vi "2. QRcode.vi"() -> ()   [LabVIEW 2019]
uses:
  <vilib>/vision/Instrument.llb/QR Code Report.ctl
  <vilib>/vision/Instrument.llb/QR Code Model Type.ctl
  <vilib>/vision/Instrument.llb/QR Code Stream Mode Type.ctl
  <vilib>/vision/Instrument.llb/Data Matrix Polarity.ctl
  <vilib>/vision/Instrument.llb/Demodulation Mode.ctl
  <vilib>/vision/Instrument.llb/Cell Sample Size.ctl
  <vilib>/vision/Instrument.llb/Cell Filter Mode.ctl
panel:
  in  "stop":bool
  out "Data":string
  out "Found?":bool
  out "QR Barcode Report (2D Barcode Reader 1)":T1={"Found?"=FALSE, "Data"="", "Bounding Box"=[], "Errors Corrected"=0, "Dimensions (Rows/Cols)"=0, "Version"=0, "QR Model"=3, "Stream Mode"=0, "Barcode Polarity"=-2, "Mirrored?"=FALSE, "Append Stream Position"=0, "Size of Append Stream"=0, "First EAN-128 ID"=0, "First Alternate Language ID"=0, "Append Stream ID"=0, "Minimum Edge Strength"=30, "Demodulation Mode"=-2, "Cell Sample Size"=-2, "Cell Filter Mode"=-2} {"Append Stream ID" format="%x"; "Cell Filter Mode" items=["Auto-detect"=-2, "Average"=0, "Median"=1, "Central Average"=2, "High Average"=3, "Low Average"=4, "Very High Average"=5, "Very Low Average"=6, "All Filters"=8]; "Cell Sample Size" items=["Auto-detect"=-2, "1x1"=1, "2x2"=2, "3x3"=3, "4x4"=4, "5x5"=5, "6x6"=6, "7x7"=7]; "Demodulation Mode" items=["Auto-detect"=-2, "Histogram"=0, "Local Contrast"=1, "Combination"=2, "All"=3]; "Barcode Polarity" items=["Auto-detect"=-2, "Black on White"=0, "White on Black"=1]; "Stream Mode" items=["Auto-detect", "Numeric", "AlphaNumeric", "Mixed", "Raw Bytes", "UCC/EAN-128 - In Tokens", "UCC/EAN-128 - In Data", "Extended Character Interpretation", "Kanji"]; "QR Model" items=["Auto Detect", "Micro", "Model 1", "Model 2"]; "Version" max=40 step=1}
  out "ORI":T8(plugin-control)
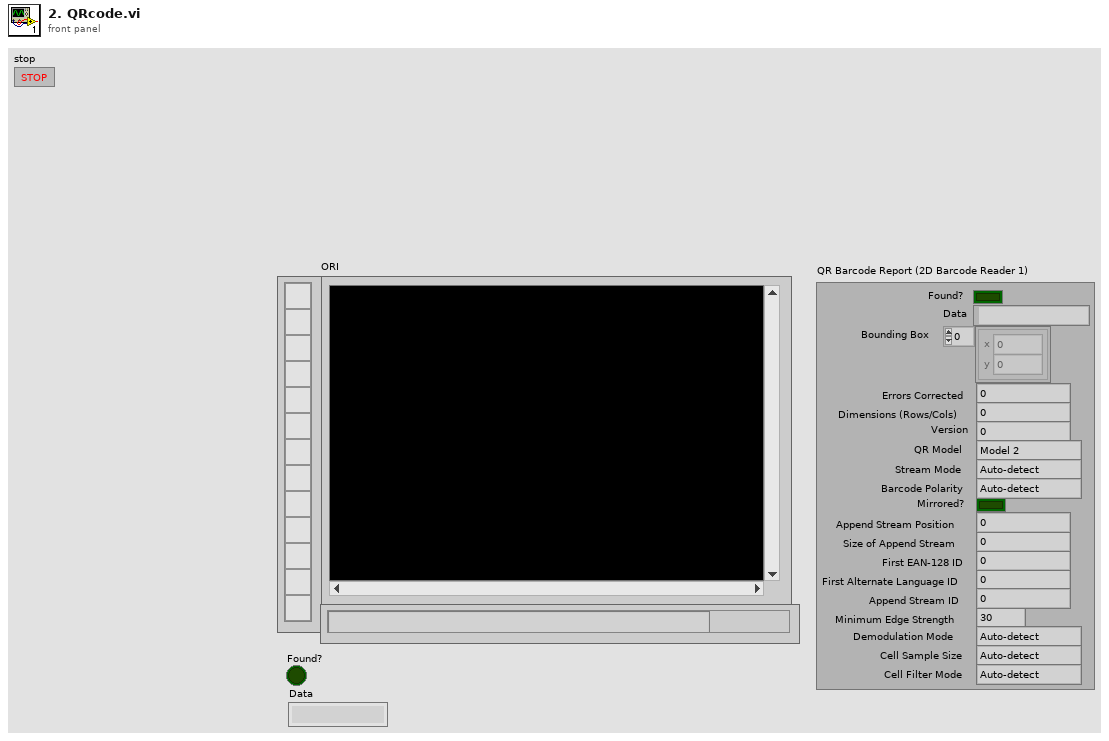
[diagram p1: front panel]
types:
  T1 = typedef "QR Code Report.ctl" = cluster{"Found?":bool, "Data":string, "Bounding Box":cluster{"x":sgl, "y":sgl}[], "Errors Corrected":u32, "Dimensions (Rows/Cols)":u32, "Version":u32, "QR Model":T2, "Stream Mode":T3, "Barcode Polarity":T4, "Mirrored?":bool, "Append Stream Position":u32, "Size of Append Stream":u32, "First EAN-128 ID":i32, "First Alternate Language ID":i32, "Append Stream ID":u32, "Minimum Edge Strength":u32, "Demodulation Mode":T5, "Cell Sample Size":T6, "Cell Filter Mode":T7}
  T2 = typedef "QR Code Model Type.ctl" = i32
  T3 = typedef "QR Code Stream Mode Type.ctl" = i32
  T4 = typedef "Data Matrix Polarity.ctl" = i32
  T5 = typedef "Demodulation Mode.ctl" = i32
  T6 = typedef "Cell Sample Size.ctl" = i32
  T7 = typedef "Cell Filter Mode.ctl" = i32
  T8 = typedef "IMAQ Image.ctl" = refnum<image>
  T9 = typedef "Image Type" = u32
  T10 = cluster{"Left":i32, "Top":i32, "Right":i32, "Bottom":i32}
  T11 = cluster{"Desired Font (Application)":enum16{"User-specified Font", "Application Font", "System Font", "Dialog Font"}, "[User-specified Font]":cluster{"Font Name":string, "Size":i16, "Strikeout?":bool, "Italic?":bool, "Underline?":bool, "Outline?":bool, "Shadow?":bool, "Bold?":bool, "Rotation Angle":dbl}, "Horizontal Alignment":i16, "Vertical Alignment":i16}
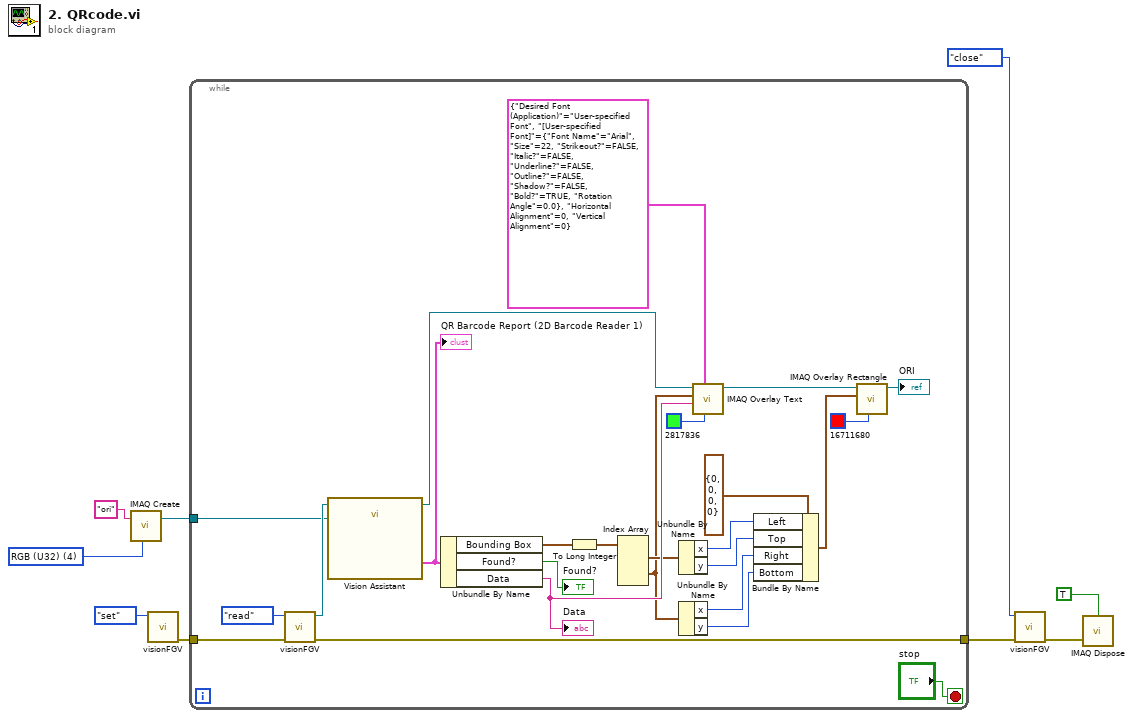
[diagram p0: block diagram]
diagram:
  w3 = T9 4 items=["Grayscale (U8)", "Grayscale (I16)", "Grayscale (SGL)", "Complex (CSG)", "RGB (U32)", "HSL (U32)", "RGB (U64)", "Grayscale (U16)"] ("Image Type")
  n1 = call "IMAQ Create"("Image Name"="ori", "Image Type"=w3) -> ("New Image"=w4:T8)  [unwired: 3 in, 1 out]
  n2 = call "visionFGV.vi"("Function"=enum16{"set", "read", "close"}."set") -> ("error out"=w6:errorcluster)  [unwired: 9 in, 1 out]
  n3 = while {
    tunnel: w6 -> [w34]
    tunnel: [w32] -> w7
    tunnel: w4 -> [w30]
    stop <- "stop" stop-if-true
    n4 = call "visionFGV.vi"("Error In"=w34, "Function"=enum16{"set", "read", "close"}."read") -> ("error out"=w32:errorcluster, "Image Out fgv"=w31:T8)  [unwired: 8 in]
    n5 = call "Vision Assistant"("Image In"=w31, "Image Dst"=w30) -> ("Image Out"=w27:T8, "QR Barcode Report (2D Barcode Reader 1)"=w29:T1)  [unwired: 23 in, 1 out]
    "QR Barcode Report (2D Barcode Reader 1)" <- w29
    n6 = Unbundle By Name(w29) -> ("Bounding Box"=w24:cluster{"x":sgl, "y":sgl}[], "Found?"=→"Found?":bool, "Data"=w26:string)
    "Data" <- w26
    n7 = To Long Integer(number=w24) -> (32bit integer=w21:cluster{"x":i32, "y":i32}[])
    n8 = Index Array(array=w21) -> (element #1=w19:cluster{"x":i32, "y":i32}, element #3=w15:cluster{"x":i32, "y":i32})  [unwired: 4 in, 2 out]
    n9 = Unbundle By Name(w19) -> ("x"=w17:i32, "y"=w16:i32)
    n10 = Unbundle By Name(w15) -> ("x"=w14:i32, "y"=w13:i32)
    n11 = call "IMAQ Overlay Text"("Text Color (black)"=u32 2817836, "Font, Size & Style"=T11 {"Desired Font (Application)"=enum."User-specified Font", "[User-specified Font]"={"Font Name"="Arial", "Size"=22, "Strikeout?"=FALSE, "Italic?"=FALSE, "Underline?"=FALSE, "Outline?"=FALSE, "Shadow?"=FALSE, "Bold?"=TRUE, "Rotation Angle"=0.0}, "Horizontal Alignment"=0, "Vertical Alignment"=0}, "String"=w26, "Origin"=w15, "Image"=w27) -> ("Image Out"=w20:T8)  [unwired: 5 in, 1 out]
    n12 = Bundle By Name(cluster=T10 {"Left"=0, "Top"=0, "Right"=0, "Bottom"=0} ("Rectangle"), "Left"=w17, "Top"=w16, "Right"=w14, "Bottom"=w13) -> (w12:T10)
    n13 = call "IMAQ Overlay Rectangle"("Color"=u32 16711680, "Rectangle"=w12, "Image"=w20) -> ("Image Out"=→"ORI":T8)  [unwired: 7 in, 1 out]
  }
  n14 = call "visionFGV.vi"("Error In"=w7, "Function"=enum16{"set", "read", "close"}."close") -> ("error out"=w2:errorcluster)  [unwired: 8 in, 1 out]
  n15 = call "IMAQ Dispose"("All Images? (No)"=TRUE, "error in (no error)"=w2) -> ()  [unwired: 4 in, 1 out]
